vi "Create Resources.vi"() -> (4 "address space collection":refnum<class "Address Space Collection.lvclass">, 15 "tx dsp":refnum<class "niUSRP Tx DSP v2 FPGA.lvclass">)   [LabVIEW 2025, in "niUSRP Tx DSP v2 FPGA.lvclass"]
uses:
  niUSRP Tx DSP v2 FPGA.lvclass
  C:/Program Files/NI/LVAddons/niidl/1/instr.lib/_niInstr/Instruction Framework/v1/FPGA/Interfaces/Address Space/Address Space.lvclass
  <instrlib>/_niInstr/Instruction Framework/v1/FPGA/Interfaces/Address Space Collection/Address Space Collection.lvclass
  niUSRP Tx DSP v2 FPGA.lvclass/niUSRP Tx DSP v2 FPGA.ctl
  <vilib>/rvi/DataTransferAndStorage/Container/Common/niFpgaContainerExecOnDevCompGetState.vi
  <vilib>/rvi/Emulation/niFpgaEmulationIsFPGAContextNoSignature.vi
  <vilib>/rvi/DataTransferAndStorage/Container/Common/niFpgaContainerGetUniqueNameForEmu.vi
  <vilib>/rvi/Memory/Memory_Emulation/niFpgaMemoryEmulationCacheClearOnFirstRun.vi
  <vilib>/rvi/Memory/Memory_Emulation/nirvimemoryEmulationManagerCache_MakeExclusive.vi
  <vilib>/rvi/Memory/Memory_Emulation/niFpgaMemoryEmulationValidateCache.vi
  <vilib>/rvi/Memory/Memory_Emulation/nirvimemoryEmulationManagerCache_InsertValue.vi
  <vilib>/Utility/error.llb/Clear Errors.vi
  <vilib>/rvi/Memory/Memory_Emulation/nirvimemoryEmulationManagerCache_ReleaseExclusive.vi
  <vilib>/rvi/Memory/Memory_Emulation/nirvimemoryEmulationManagerCache_GetValue.vi
  <vilib>/rvi/Memory/Memory_Emulation/nirvimemoryEmulationManagerCache_SetValue.vi
  <vilib>/rvi/Emulation/niFpgaProcessEmulError.vi
  <vilib>/rvi/Emulation/niFpgaSctlEmulationGetInTimedLoop.vi
  <vilib>/rvi/DataTransferAndStorage/Container/XNode/niFpgaContainer.xnode
  <vilib>/rvi/DataTransferAndStorage/Register/Emulation/niFpgaRegisterEmulationRefIn.vi
  <instrlib>/_niInstr/Basic Elements/v1/FPGA/niInstr Basic Elements v1 FPGA.lvlib
  <instrlib>/_niInstr/Instruction Framework/v1/FPGA/Collection Builder/Collection Builder.lvclass
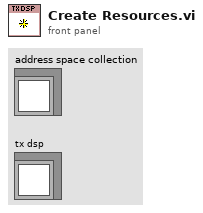
[diagram p1: front panel]
types:
  T1 = typedef "niInstr Address Space Collection Builder v1 FPGA.lvlib/Parent Metadata.ctl" = cluster{"UID":u16, "version":u16, "oldest compatible version":u16}
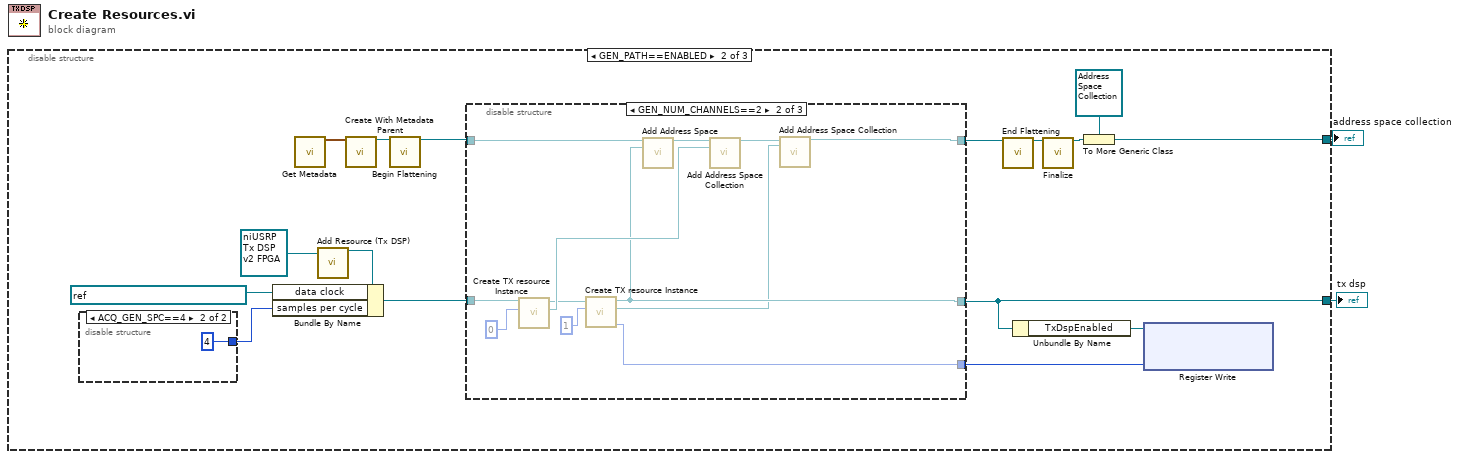
[diagram p0: block diagram]
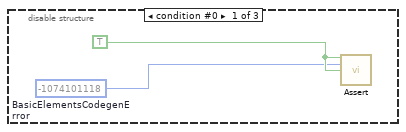
[diagram p2: hidden frame]
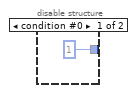
[diagram p3: hidden frame]
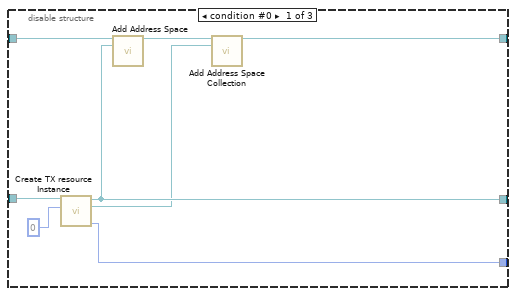
[diagram p4: hidden frame]
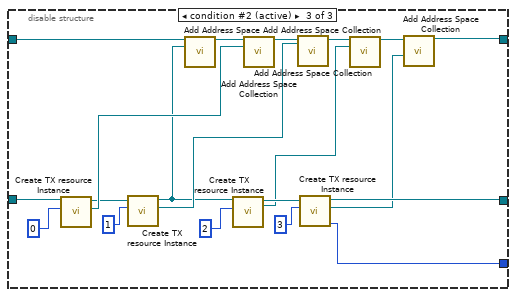
[diagram p5: hidden frame]
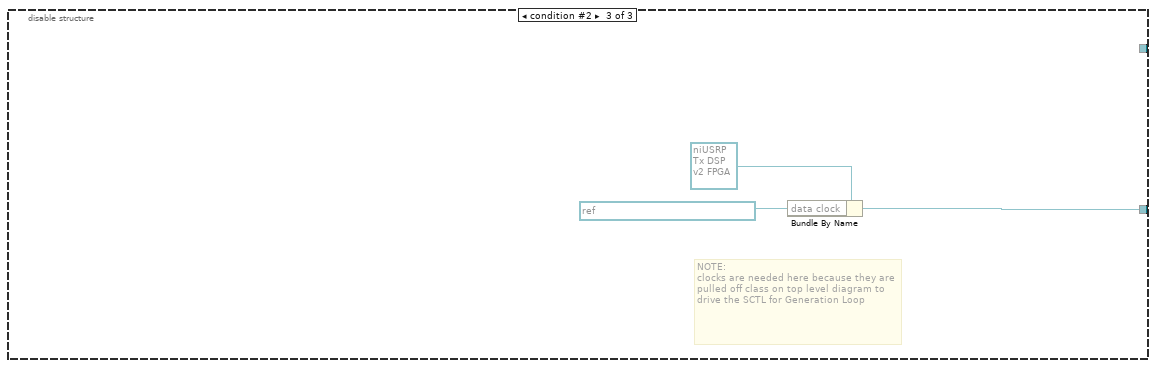
[diagram p6: hidden frame]
diagram:
  n1 = disable-structure shown="GEN_PATH==ENABLED" {
    disable-tunnel: [_ w7 w63] -> w2
    disable-tunnel: [_ w14 _] -> w1
    frame condition #0 {
      w4 = TRUE ("assert")
      w3 = -1074101118  # BasicElementsCodegenError
      n2 = call <instrlib>:"Assert.vi"("assert"=w4, "error code"=w3, "enable show error"=w4) -> ()  [unwired: 13 in]
    }
    frame condition #1 (active) {
      n3 = disable-structure shown="ACQ_GEN_SPC==4" {
        disable-tunnel: [u16 1 ("samples per cycle (SPC)") u16 4 ("samples per cycle (SPC)")] -> w8
        frame condition #0 {
        }
        frame condition #1 (active) {
        }
      }
      n4 = call "Get Metadata.vi"() -> ("gen metadata"=w20:T1)  [unwired: 15 in]
      n5 = call "Add Resource (Tx DSP).vi"("niUSRP Tx DSP v2 FPGA.lvclass"=refnum<class "niUSRP Tx DSP v2 FPGA.lvclass"> refnum ("gen in")) -> ("niUSRP Tx DSP v2 FPGA.lvclass 2"=w12:refnum<class "niUSRP Tx DSP v2 FPGA.lvclass">)  [unwired: 14 in]
      n6 = Bundle By Name(cluster=w12, "data clock"=refnum<k21> "Daughterboard 0\\DataClock" ("clock x2"), "samples per cycle"=w8) -> (w15:refnum<class "niUSRP Tx DSP v2 FPGA.lvclass">)
      n7 = call <instrlib>:"Create With Metadata Parent.vi"("parent metadata"=w20) -> ("collection builder"=w19:refnum<class "Collection Builder.lvclass">)  [unwired: 14 in]
      n8 = call <instrlib>:"Begin Flattening.vi"("collection builder in"=w19) -> ("collection builder out"=w10:refnum<class "Collection Builder.lvclass">)  [unwired: 14 in]
      n9 = disable-structure shown="GEN_NUM_CHANNELS==2" {
        disable-tunnel: w15 -> [w30 w42 w62]
        disable-tunnel: [w29 w34 w49] -> w7
        disable-tunnel: w10 -> [w27 w40 w60]
        disable-tunnel: [w25 w36 w46] -> w9
        disable-tunnel: [w23 w31 w43] -> w5
        frame condition #0 {
          n10 = call "Create TX resource Instance.vi"("instance"=u8 0, "niUSRP Tx DSP v2 FPGA in"=w30) -> ("TxDspEnabled"=w23:u64, "address space collection"=w24:refnum<class "Address Space Collection.lvclass">, "niUSRP Tx DSP v2 FPGA out"=w29:refnum<class "niUSRP Tx DSP v2 FPGA.lvclass">)  [unwired: 7 in]
          n11 = call <instrlib>:"Add Address Space.vi"("collection builder in"=w27, "address space"=w29) -> ("collection builder out"=w26:refnum<class "Collection Builder.lvclass">)  [unwired: 13 in]
          n12 = call <instrlib>:"Add Address Space Collection.vi"("collection builder in"=w26, "address space collection"=w24) -> ("collection builder out"=w25:refnum<class "Collection Builder.lvclass">)  [unwired: 13 in]
        }
        frame condition #1 {
          n13 = call "Create TX resource Instance.vi"("instance"=u8 0, "niUSRP Tx DSP v2 FPGA in"=w42) -> ("address space collection"=w38:refnum<class "Address Space Collection.lvclass">, "niUSRP Tx DSP v2 FPGA out"=w35:refnum<class "niUSRP Tx DSP v2 FPGA.lvclass">)  [unwired: 7 in, 1 out]
          n14 = call "Create TX resource Instance.vi"("instance"=u8 1, "niUSRP Tx DSP v2 FPGA in"=w35) -> ("TxDspEnabled"=w31:u64, "address space collection"=w33:refnum<class "Address Space Collection.lvclass">, "niUSRP Tx DSP v2 FPGA out"=w34:refnum<class "niUSRP Tx DSP v2 FPGA.lvclass">)  [unwired: 7 in]
          n15 = call <instrlib>:"Add Address Space.vi"("collection builder in"=w40, "address space"=w34) -> ("collection builder out"=w39:refnum<class "Collection Builder.lvclass">)  [unwired: 13 in]
          n16 = call <instrlib>:"Add Address Space Collection.vi"("collection builder in"=w39, "address space collection"=w38) -> ("collection builder out"=w37:refnum<class "Collection Builder.lvclass">)  [unwired: 13 in]
          n17 = call <instrlib>:"Add Address Space Collection.vi"("collection builder in"=w37, "address space collection"=w33) -> ("collection builder out"=w36:refnum<class "Collection Builder.lvclass">)  [unwired: 13 in]
        }
        frame condition #2 (active) {
          n18 = call "Create TX resource Instance.vi"("instance"=u8 0, "niUSRP Tx DSP v2 FPGA in"=w62) -> ("address space collection"=w58:refnum<class "Address Space Collection.lvclass">, "niUSRP Tx DSP v2 FPGA out"=w56:refnum<class "niUSRP Tx DSP v2 FPGA.lvclass">)  [unwired: 7 in, 1 out]
          n19 = call "Create TX resource Instance.vi"("instance"=u8 1, "niUSRP Tx DSP v2 FPGA in"=w56) -> ("address space collection"=w54:refnum<class "Address Space Collection.lvclass">, "niUSRP Tx DSP v2 FPGA out"=w50:refnum<class "niUSRP Tx DSP v2 FPGA.lvclass">)  [unwired: 7 in, 1 out]
          n20 = call <instrlib>:"Add Address Space.vi"("collection builder in"=w60, "address space"=w50) -> ("collection builder out"=w59:refnum<class "Collection Builder.lvclass">)  [unwired: 13 in]
          n21 = call "Create TX resource Instance.vi"("instance"=u8 2, "niUSRP Tx DSP v2 FPGA in"=w50) -> ("address space collection"=w45:refnum<class "Address Space Collection.lvclass">, "niUSRP Tx DSP v2 FPGA out"=w52:refnum<class "niUSRP Tx DSP v2 FPGA.lvclass">)  [unwired: 7 in, 1 out]
          n22 = call <instrlib>:"Add Address Space Collection.vi"("collection builder in"=w59, "address space collection"=w58) -> ("collection builder out"=w57:refnum<class "Collection Builder.lvclass">)  [unwired: 13 in]
          n23 = call <instrlib>:"Add Address Space Collection.vi"("collection builder in"=w57, "address space collection"=w54) -> ("collection builder out"=w47:refnum<class "Collection Builder.lvclass">)  [unwired: 13 in]
          n24 = call "Create TX resource Instance.vi"("instance"=u8 3, "niUSRP Tx DSP v2 FPGA in"=w52) -> ("TxDspEnabled"=w43:u64, "address space collection"=w44:refnum<class "Address Space Collection.lvclass">, "niUSRP Tx DSP v2 FPGA out"=w49:refnum<class "niUSRP Tx DSP v2 FPGA.lvclass">)  [unwired: 7 in]
          n25 = call <instrlib>:"Add Address Space Collection.vi"("collection builder in"=w47, "address space collection"=w45) -> ("collection builder out"=w48:refnum<class "Collection Builder.lvclass">)  [unwired: 13 in]
          n26 = call <instrlib>:"Add Address Space Collection.vi"("collection builder in"=w48, "address space collection"=w44) -> ("collection builder out"=w46:refnum<class "Collection Builder.lvclass">)  [unwired: 13 in]
        }
      }
      n27 = call <instrlib>:"End Flattening.vi"("collection builder in"=w9) -> ("collection builder out"=w17:refnum<class "Collection Builder.lvclass">)  [unwired: 14 in]
      n28 = Unbundle By Name(w7) -> ("TxDspEnabled"=w6:refnum<k21>)
      n29 = call <instrlib>:"Finalize.vi"("collection builder in"=w17) -> ("address space collection"=w16:refnum<class "Address Space Collection.lvclass">)  [unwired: 14 in]
      n30 = To More Generic Class(target class=refnum<class "Address Space Collection.lvclass"> refnum ("collection"), reference=w16) -> (generic class reference=w14:refnum<class "Address Space Collection.lvclass">)
      n31 = xnode "Register Write"("Data"=w5, "Register In"=w6) -> ()  [unwired: 1 out]
    }
    frame condition #2 {
      # "NOTE:\nclocks are needed here because they are pulled off class on top level diagram to drive the SCTL for Generation Loop"
      n32 = Bundle By Name(cluster=refnum<class "niUSRP Tx DSP v2 FPGA.lvclass"> refnum ("gen"), "data clock"=refnum<k21> "Daughterboard 0\\DataClock") -> (w63:refnum<class "niUSRP Tx DSP v2 FPGA.lvclass">)
    }
  }
  "tx dsp" <- w2
  "address space collection" <- w1
